vi "Make sequential file name.vi"(2 "Serial number":i32, 3 "File name information":T1) -> (0 "Path out":path)   [LabVIEW 2011]
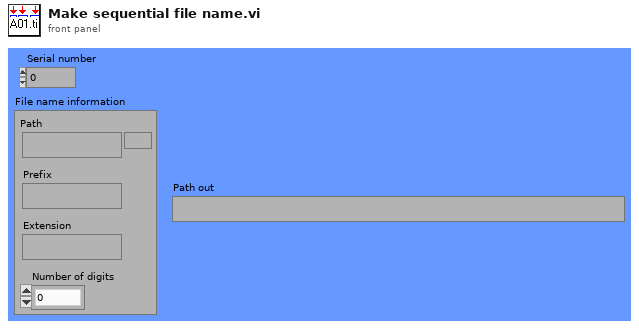
[diagram p1: front panel]
types:
  T1 = cluster{"Path":path, "Prefix":string, "Extension":string, "Number of digits":i32}
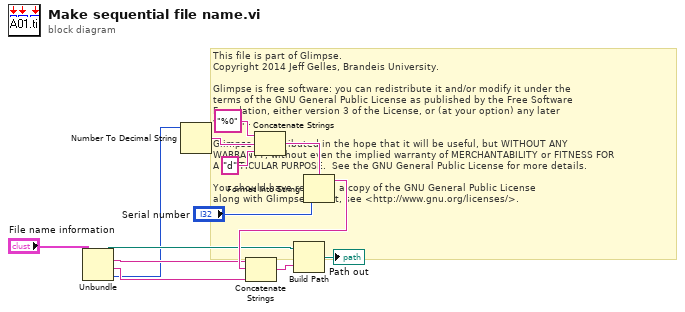
[diagram p0: block diagram]
diagram:
  # "This file is part of Glimpse. \nCopyright 2014 Jeff Gelles, Brandeis University.    \n\nGlimpse is free software: you can redistribute it and/or modify it under the \nterms of the GNU General Public License as published by the Free Software \nFoundation, either version 3 of the License, or (at your option) any later \nversion.\n\nGlimpse is distributed in the hope that it will be useful, but WITHOUT ANY \nWARRANTY; without even the implied warranty of MERCHANTABILITY or FITNESS FOR \nA PARTICULAR PURPOSE.  See the GNU General Public License for more details.\n\nYou should have received a copy of the GNU General Public License\nalong with Glimpse.  If not, see <http://www.gnu.org/licenses/>."
  n1 = Unbundle("File name information") -> ("Path"=w9:path, "Prefix"=w10:string, "Extension"=w12:string, "Number of digits"=w1:i32)
  n2 = Number To Decimal String(number=w1) -> (decimal integer string=w3:string)  [unwired: 1 out]
  n3 = Concatenate Strings("%0" ("Substring"), w3, "d" ("Substring")) -> (w6:string)
  n4 = Format Into String(format string=w6, "Serial number") -> (resulting string=w11:string)  [unwired: 2 in, 1 out]
  n5 = Concatenate Strings(w10, w11, w12) -> (w7:string)
  n6 = Build Path(base path=w9, name or relative path=w7) -> (appended path=→"Path out":path)
